vi "Save column names.vi"(8 "error in (no error)":errorcluster, 10 "Save data details":T1) -> (0 "error out":errorcluster, 2 "Save data details out":T1)   [LabVIEW 2015]
uses:
  Controls/Save data details.ctl
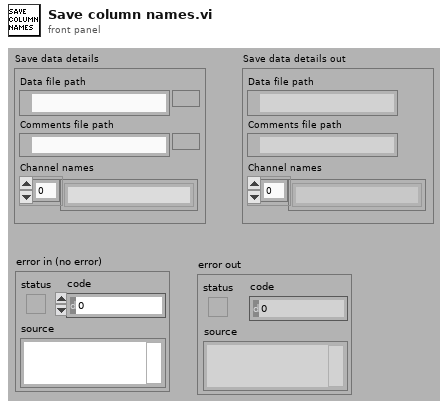
[diagram p1: front panel]
types:
  T1 = typedef "Save data details.ctl" = cluster{"Data file path":path, "Comments file path":path, "Channel names":string[]}
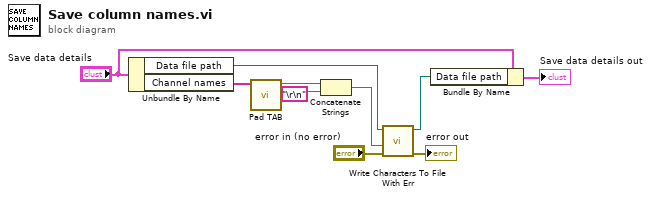
[diagram p0: block diagram]
diagram:
  n1 = Unbundle By Name("Save data details") -> ("Data file path"=w10:path, "Channel names"=w9:string[])
  n2 = call "Pad TAB.vi"("Input String Array"=w9) -> ("Output String"=w8:string)  [unwired: 1 in, 9 out]
  n3 = Concatenate Strings(w8, "\r\n") -> (w7:string)
  n4 = call "Write Characters To File With Err.vi"("error in (no error)"="error in (no error)", "character string"=w7, "file path (dialog if empty)"=w10) -> ("error out"=→"error out":errorcluster, "new file path (Not A Path if cancelled)"=w4:path)  [unwired: 2 in, 5 out]
  n5 = Bundle By Name(cluster="Save data details", "Data file path"=w4) -> (→"Save data details out":T1)
